vi "Doppler Moving STFT PtByPt Rev1.vi"() -> ()   [LabVIEW 2022 SP3]
doc: "Performs real-time Joint Time Frequency Analysis (JTFA) using Point By Point STFT. The signal is simulated by a sine wave plus Gaussian noise."
uses:
  <vilib>/measure/mamon.llb/Waveform Peak Detection for N Chan.vi
  <vilib>/measure/mascope.llb/Pulse Measurements 1 chan.vi
  <vilib>/ptbypt/NI_PtbyPt.lvlib
  <vilib>/measure/NI_MAPro.lvlib
panel:
  out "period 2":dbl
  out "period":dbl
  out "Waveform Graph 4":dynamicdata(graph)
  out "Waveform Graph 3":dbl[](graph)
  out "Waveform Graph 2":dbl[](graph)
  out "locations time 1":dbl[](array[numeric])
  out "locations time 0":dbl[](array[numeric])
  out "Locations":cluster{"Locations":dbl[]}[](array[cluster]) {"Locations" format="%.2p"}
  out "Amplitudes":cluster{"Amplitudes":dbl[]}[](array[cluster]) {"Amplitudes" format="%.2p"}
  out "# peaks found":i32[](array[numeric])
  out "Waveform Graph":dbl[][](graph)
  out "Array 3":dbl[][](array[numeric])
  out "DT":dbl
  out "dt":dbl
  out "Number of cols (freq)":dbl
  out "Number of rows (time)":dbl
  out "Array 2":i32[](array[numeric])
  in  "time increment":i32=200
  out "Doppler signal":dynamicdata(graph) caption="Signals"
  out "Moving STFT":dbl[][](graph)
  in  "sample length":i32=200
  in  "window length":i32=100 format="%0.0f"
  in  "stop":bool
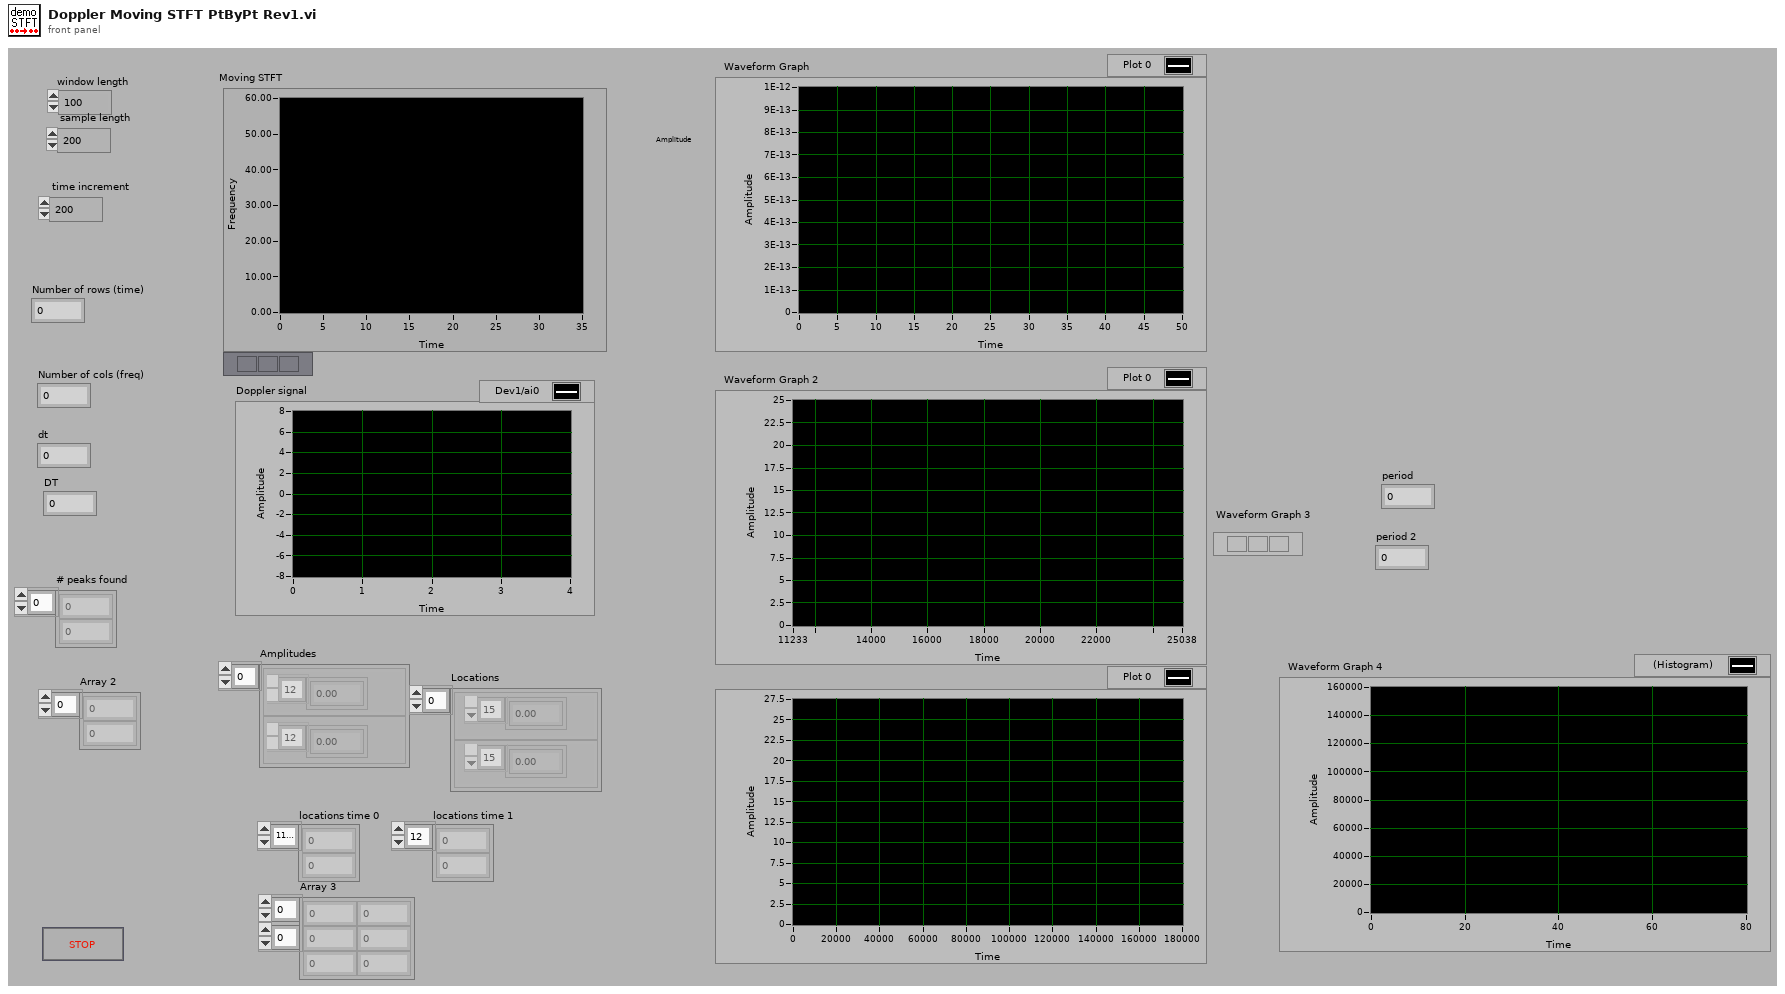
[diagram p1: front panel]
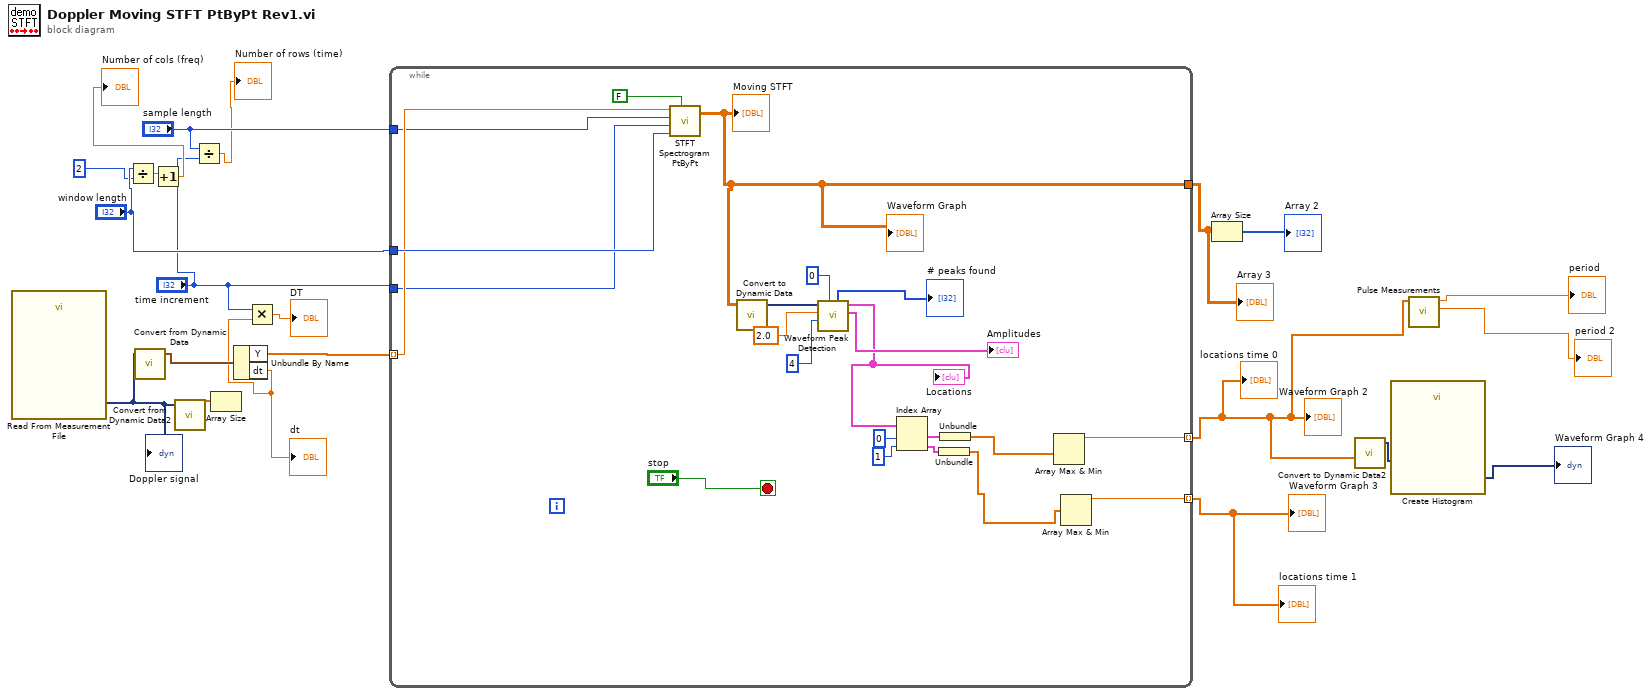
[diagram p0: block diagram]
diagram:
  n1 = call "Read From Measurement File"() -> ("Signals"=w18:dynamicdata)  [unwired: 4 in, 7 out]
  "Doppler signal" <- w18
  n2 = Divide(x="window length", y=u32 2 ("milliseconds to wait")) -> (x/y=w14:dbl)
  n3 = call "Convert from Dynamic Data"("Dynamic Data Type"=w18) -> ("Waveform"=w19:waveform(dbl))  [unwired: 1 in, 2 out]
  n4 = Increment(x=w14) -> (x+1=→"Number of cols (freq)":dbl)
  n5 = call "Convert from Dynamic Data2"("Dynamic Data Type"=w18) -> ("Array"=w17:dbl[])  [unwired: 3 out]
  n6 = Divide(x="sample length", y="time increment") -> (x/y=→"Number of rows (time)":dbl)
  n7 = Array Size(array=w17) -> ()  [unwired: 1 out]
  n8 = Unbundle By Name(w19) -> ("Y"=w21:dbl[], "dt"=w8:dbl)
  "dt" <- w8
  n9 = Multiply(x="time increment", y=w8) -> (x*y=→"DT":dbl)
  n10 = while {
    tunnel: "window length" -> [w43]
    tunnel: w21 -> [w42] mode=indexing
    tunnel: "time increment" -> [w41]
    tunnel: "sample length" -> [w40]
    tunnel: [w38] -> w7
    tunnel: [w24] -> w3 mode=indexing
    tunnel: [w23] -> w6 mode=indexing
    stop <- "stop" stop-if-true
    n11 = call <vilib>:"STFT Spectrogram PtByPt.vi"("initialize"=FALSE, "window length"=w43, "time increment"=w41, "sample length"=w40, "x"=w42) -> ("STFT Spectrogram {X}"=w38:dbl[][])  [unwired: 1 in, 1 out]
    "Moving STFT" <- w38
    "Waveform Graph" <- w38
    n12 = call "Convert to Dynamic Data"("2D Array"=w38) -> ("Dynamic Data Type"=w37:dynamicdata)  [unwired: 3 out]
    n13 = call-poly <vilib>:"Waveform Peak Detection.vi"("peaks/valleys"=u32 0 ("milliseconds to wait"), "width"=u32 4 ("milliseconds to wait"), "threshold"=2.0 ("Y Scale.Range:Minimum"), "Signals In"=w37) -> ("Amplitudes"=→"Amplitudes":cluster{"Amplitudes":dbl[]}[], "Locations"=w31:cluster{"Locations":dbl[]}[], "# found"=→"# peaks found":i32[])  [unwired: 3 in, 2 out]
    "Locations" <- w31
    n14 = Index Array(array=w31, index #1=u32 0 ("milliseconds to wait"), index #2=u32 1 ("milliseconds to wait")) -> (element #1=w29:cluster{"Locations":dbl[]}, element #2=w27:cluster{"Locations":dbl[]})
    n15 = Unbundle(w27) -> ("Locations"=w25:dbl[])
    n16 = Unbundle(w29) -> ("Locations"=w26:dbl[])
    n17 = Array Max & Min(array=w26) -> (max value=w24:dbl)  [unwired: 3 out]
    n18 = Array Max & Min(array=w25) -> (max value=w23:dbl)  [unwired: 3 out]
  }
  "Array 3" <- w7
  "Waveform Graph 2" <- w3
  "Waveform Graph 3" <- w6
  "locations time 0" <- w3
  "locations time 1" <- w6
  n19 = Array Size(array=w7) -> (size(s)=→"Array 2":i32[])
  n20 = call "Convert to Dynamic Data2"("Array"=w3) -> ("Dynamic Data Type"=w5:dynamicdata)  [unwired: 3 out]
  n21 = call "Create Histogram"("Signal"=w5) -> ("Histogram"=→"Waveform Graph 4":dynamicdata)  [unwired: 3 in, 7 out]
  n22 = call-poly <vilib>:"Pulse Measurements.vi"("signal in"=w3) -> ("pulse duration"=→"period 2":dbl, "period"=→"period":dbl)  [unwired: 3 in, 6 out]
